vi "Realign uSs from Run Config.vi"(8 "error in (no error)":errorcluster, 10 "uS List":string[](array[string]), 11 "Guardian in":refnum<class "Guardian.lvclass">) -> (0 "error out":errorcluster, 3 "Guardian out":refnum<class "Guardian.lvclass">)   [LabVIEW 2026, in "TALOS.lvlib" / "Guardian.lvlib" / "Guardian.lvclass"]
uses:
  Guardian.lvclass
  C:/LabVIEW Code/TALOS/builds/Actor Framework PPL/Actor Framework.lvlibp/1abvi3w/vi.lib/ActorFramework/Actor/Actor.lvclass
  Classes/uService List/uService List.lvclass/uService List.ctl
  Guardian Messages/Kill uService Msg/Kill uService Msg.lvclass/Kill uService Msg.ctl
  Guardian Messages/Launch uService Msg/Launch uService Msg.lvclass/Launch uService Msg.ctl
  Ancestor/Ancestor/Ancestor.lvclass/Ancestor.ctl
  Classes/uService List/Get all IDs.vi
  fcb3572a-2cec-4fc7-ae89-858ca11508d7.vi
  24f5ad44-0365-4765-b898-cef69fd9b7bb.vi
  Support VIs/Generate Error.vi
  FGV/Error Memory/Get Error Description.vi
  Support VIs/Get PC name.vi
  Ancestor/Ancestor/Read ID.vi
  Support VIs/Get Class Name.vi
  <vilib>/Utility/error.llb/Clear Errors.vi
  FGV/Error Memory/Error Memory Core.vi
  <vilib>/AdvancedString/Delimited String to 1D String Array.vi
  <vilib>/AdvancedString/Delimited String to 1D String Array (string).vi
  Support VIs/Circus Root Path.vi
  FGV/Error Memory/Error Crt Lvl checker.vi
  FGV/Error Memory/Error Memory Core.vi/40c8088d-b597-4017-91af-faa98e00292e.vi
  FGV/Error Memory/Error Memory Core.vi/d4a3ab98-063c-4e44-b43d-fbdcfe6c2be2.vi
  Support VIs/Global Constants.vi
  builds/Actor Framework PPL/Actor Framework.lvlibp/1abvi3w/vi.lib/ActorFramework/Message Enqueuer/Enqueue.vi
  Support VIs/Global Memory.vi
  <vilib>/Utility/LVClass/Get LV Class Name.vi
  Support VIs/Is in Packed Library.vi
  Support VIs/TALOS Root path.vi
  Support VIs/Read CSV worksheet.vi
  <vilib>/Utility/error.llb/General Error Handler.vi
  Support VIs/Error Log.vi
  Guardian Messages/Kill uService Msg/Kill uService Msg.lvclass
  Guardian Messages/Launch uService Msg/Launch uService Msg.lvclass
  Guardian Messages/I am alive Msg/I am alive Msg.lvclass
  Ancestor/Ancestor/Ancestor.lvclass
  <vilib>/Comparison/Equal/Equal Functor/Equal Functor.lvclass
  Classes/uService List/uService List.lvclass
  builds/Actor Framework PPL/Actor Framework.lvlibp/1abvi3w/vi.lib/ActorFramework/Actor/Actor.lvclass
  TALOS.lvlib
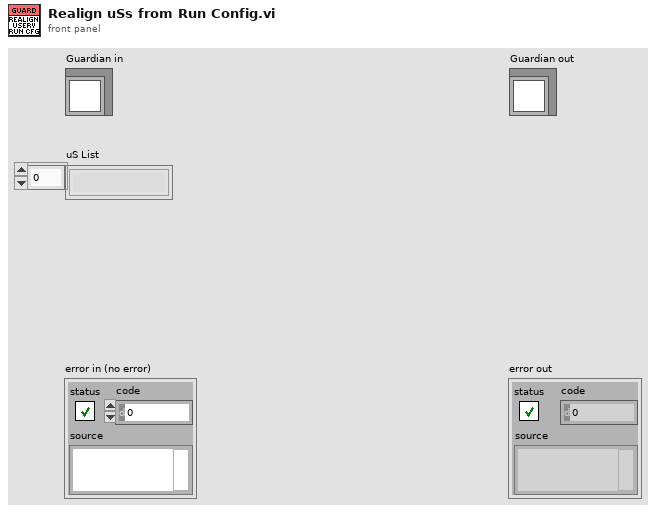
[diagram p1: front panel]
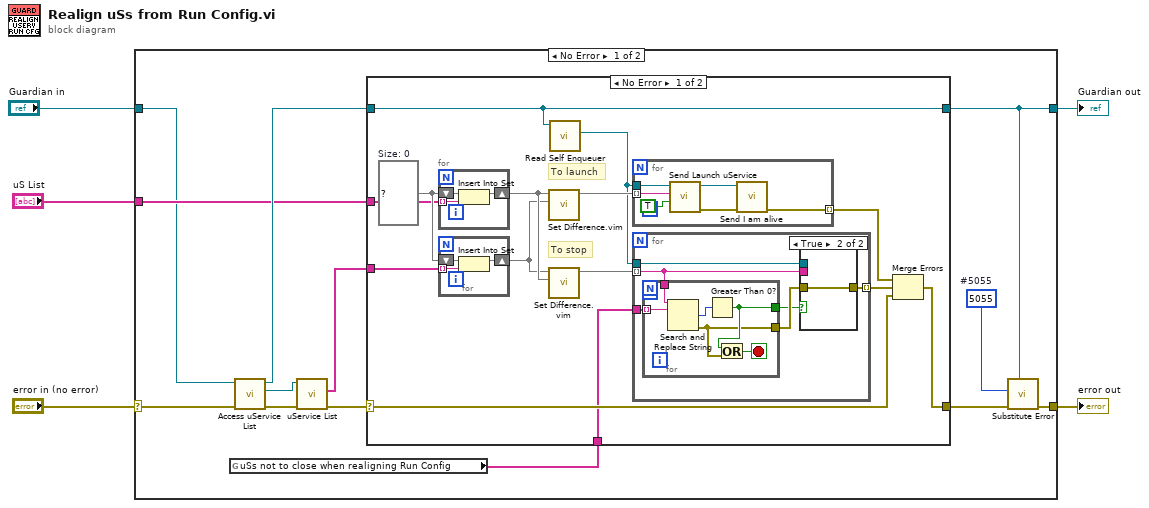
[diagram p0: block diagram]
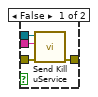
[diagram p2: hidden frame]
diagram:
  n1 = case shown="No Error" "error in (no error)" {
    selector: "error in (no error)" -> [w8 w65]
    tunnel: [w12 w65] -> w4
    tunnel: [w11 w64] -> w2
    tunnel: "Guardian in" -> [w6 w64]
    tunnel: "uS List" -> [w7 _]
    frame No Error {
      w10 = 5055  # #5055
      n2 = global read "Global Constants.vi" "uSs not to close when realigning Run Config"() -> (w9:string[])
      n3 = call-dynamic "Access uService List.vi"("error in (no error)"=w8, "Ancestor in"=w6) -> ("error out"=w17:errorcluster, "uService List out"=w18:refnum<class "uService List.lvclass">, "Ancestor out"=w15:refnum<class "Guardian.lvclass">)  [unwired: 7 in]
      n4 = call-poly "uService List.vi"("error in (no error)"=w17, "uService List"=w18) -> ("error out"=w14:errorcluster, "All IDs"=w16:string[])  [unwired: 7 in, 1 out]
      n5 = case shown="No Error" w14 {
        selector: w14 -> [w21 w63]
        tunnel: w7 -> [w29 _]
        tunnel: w16 -> [w27 _]
        tunnel: w15 -> [w25 w62]
        tunnel: [w20 w63] -> w13
        tunnel: [w25 w62] -> w11
        tunnel: w9 -> [w19 _]
        frame No Error {
          w30 = set{string} {}  # Size: 0
          # "To stop"
          # "To launch"
          n6 = for {
            shift-right: [w38] -> w28
            shift-left: w30 -> [w37]
            tunnel: w29 -> [w36] mode=indexing
            n7 = Insert Into Set(10:w36, 11:w37) -> (3:w38:set{string})  [unwired: 1 out]
          }
          n8 = for {
            shift-right: [w35] -> w26
            shift-left: w30 -> [w34]
            tunnel: w27 -> [w33] mode=indexing
            n9 = Insert Into Set(10:w33, 11:w34) -> (3:w35:set{string})  [unwired: 1 out]
          }
          n10 = call "Set Difference.vim"("set 2"=w26, "set 1"=w28) -> ("difference"=w32:set{string})  [unwired: 9 in]
          n11 = call "Set Difference.vim"("set 2"=w28, "set 1"=w26) -> ("difference"=w31:set{string})  [unwired: 9 in]
          n12 = call "Read Self Enqueuer.vi"("Actor"=w25) -> ("Self Enqueuer"=w24:refnum<class "Message Enqueuer.lvclass">)  [unwired: 10 in]
          n13 = for {
            tunnel: w32 -> [w60] mode=indexing
            tunnel: w24 -> [w61]
            tunnel: [w57] -> w23 mode=indexing
            n14 = call "Send Launch uService.vi"("GUI?"=TRUE, "uService Class Name"=w60, "Message Enqueuer"=w61) -> ("error out"=w58:errorcluster, "Message Enqueuer out"=w56:refnum<class "Message Enqueuer.lvclass">)  [unwired: 7 in]
            n15 = call "Send I am alive.vi"("error in (no error)"=w58, "Message Enqueuer"=w56) -> ("error out"=w57:errorcluster)  [unwired: 8 in, 1 out]
          }
          n16 = for {
            tunnel: w31 -> [w42] mode=indexing
            tunnel: w24 -> [w44]
            tunnel: [w43] -> w22 mode=indexing
            tunnel: w19 -> [w41]
            n17 = for {
              tunnel: w42 -> [w55]
              tunnel: w41 -> [w54] mode=indexing
              tunnel: [w51] -> w40
              tunnel: [w52] -> w39
              stop <- w50 stop-if-true
              n18 = Search and Replace String(input string=w55, search string=w54) -> (number of replacements=w53:i32, error out=w51:errorcluster)  [unwired: 6 in, 2 out]
              n19 = Greater Than 0?(x=w53) -> (x > 0?=w52:bool)
              n20 = Or(x=w52, y=w51) -> (x .or. y?=w50:bool)
            }
            n21 = case shown="True" w39 {
              tunnel: w44 -> [w48 _]
              tunnel: [w47 w49] -> w43
              tunnel: w42 -> [w46 _]
              tunnel: w40 -> [w45 w49]
              frame False {
                n22 = call "Send Kill uService.vi"("error in (no error)"=w45, "uService"=w46, "Message Enqueuer"=w48) -> ("error out"=w47:errorcluster)  [unwired: 7 in, 1 out]
              }
              frame True {
              }
            }
          }
          n23 = Merge Errors(w23, w22, w21) -> (w20:errorcluster)
        }
        frame Error {
        }
      }
      n24 = call "Substitute Error.vi"("LabVIEW Object"=w11, "error in (no error)"=w13, "Error Code"=w10) -> ("error out"=w12:errorcluster)  [unwired: 8 in]
    }
    frame Error {
    }
  }
  "error out" <- w4
  "Guardian out" <- w2
